vi "Calc sensitivity.vi"(7 "dB Reference":dbl=84.0, 9 "Frequency list Adjusted":T1(array[cluster])=[{"frequency [Hz]"=200.0, "amplitude [V]"=0.5}, {"frequency [Hz]"=224.0, "amplitude [V]"=0.5}, {"frequency [Hz]"=250.0, "amplitude [V]"=0.5}, {"frequency [Hz]"=280.0, "amplitude [V]"=0.5}, {"frequency [Hz]"=315.0, "amplitude [V]"=0.5}, {"frequency [Hz]"=355.0, "amplitude [V]"=0.5}, {"frequency [Hz]"=400.0, "amplitude [V]"=0.5}, {"frequency [Hz]"=450.0, "amplitude [V]"=0.5}, {"frequency [Hz]"=500.0, "amplitude [V]"=0.5}, {"frequency [Hz]"=560.0, "amplitude [V]"=0.5}, {"frequency [Hz]"=630.0, "amplitude [V]"=0.5}, {"frequency [Hz]"=710.0, "amplitude [V]"=0.5}, {"frequency [Hz]"=800.0, "amplitude [V]"=0.5}, {"frequency [Hz]"=900.0, "amplitude [V]"=0.5}, {"frequency [Hz]"=1000.0, "amplitude [V]"=0.5}, {"frequency [Hz]"=1120.0, "amplitude [V]"=0.5}, {"frequency [Hz]"=1250.0, "amplitude [V]"=0.5}, {"frequency [Hz]"=1400.0, "amplitude [V]"=0.5}, {"frequency [Hz]"=1600.0, "amplitude [V]"=0.5}, {"frequency [Hz]"=1800.0, "amplitude [V]"=0.5}, {"frequency [Hz]"=2000.0, "amplitude [V]"=0.5}, {"frequency [Hz]"=2240.0, "amplitude [V]"=0.5}, {"frequency [Hz]"=2500.0, "amplitude [V]"=0.5}, {"frequency [Hz]"=2800.0, "amplitude [V]"=0.5}, {"frequency [Hz]"=3150.0, "amplitude [V]"=0.5}, {"frequency [Hz]"=3550.0, "amplitude [V]"=0.5}, {"frequency [Hz]"=4000.0, "amplitude [V]"=0.5}, {"frequency [Hz]"=4500.0, "amplitude [V]"=0.5}, {"frequency [Hz]"=5000.0, "amplitude [V]"=0.5}, {"frequency [Hz]"=5600.0, "amplitude [V]"=0.5}, {"frequency [Hz]"=6300.0, "amplitude [V]"=0.5}, {"frequency [Hz]"=7100.0, "amplitude [V]"=0.5}, {"frequency [Hz]"=8000.0, "amplitude [V]"=0.5}] {"amplitude [V]" format="%.6f"; "frequency [Hz]" format="%.2f"}, 10 "Frequency [Hz]":dbl, 11 "Fundamental Response":T2(graph) caption="Fundamental-Response") -> (1 "Sensitivity_Pointer":i32, 2 "Sensitivity Frequency (Hz)":dbl, 3 "Sensitivity (mV/Pa)":dbl)   [LabVIEW 2018]
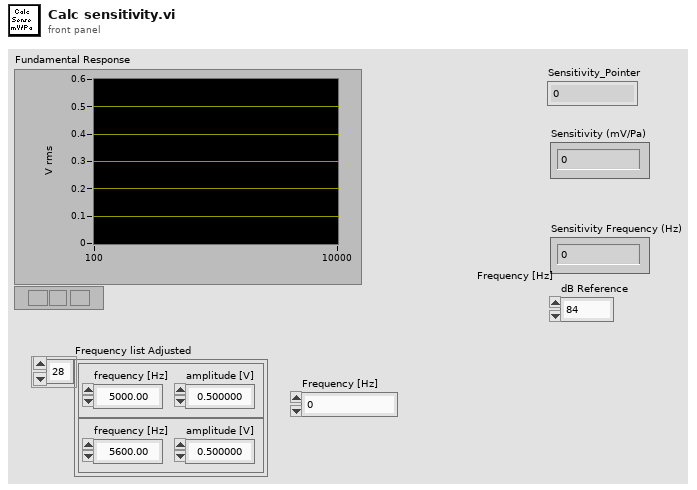
[diagram p1: front panel]
types:
  T1 = cluster{"frequency [Hz]":dbl, "amplitude [V]":dbl}[]
  T2 = cluster{"frequency [Hz]":dbl[], "amplitude":dbl[]}
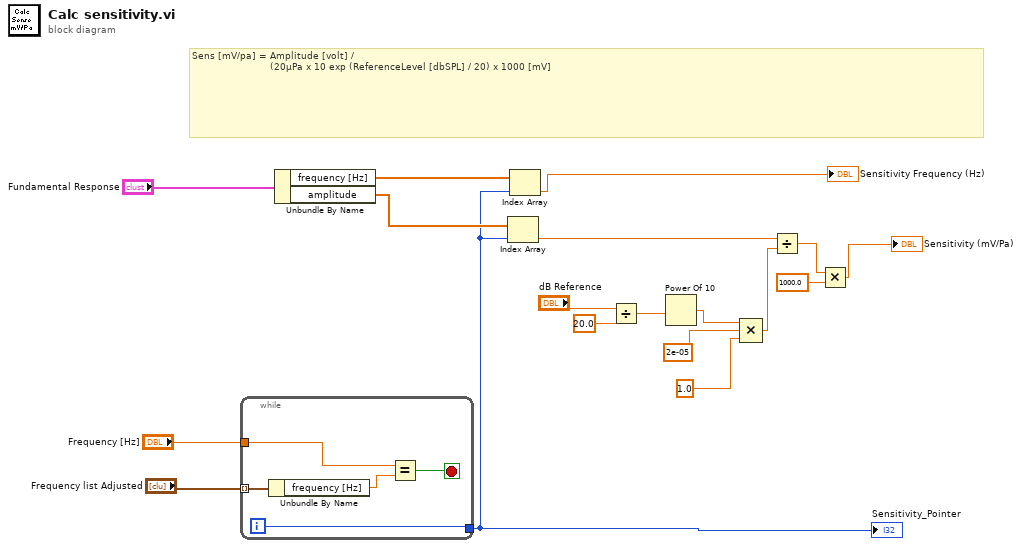
[diagram p0: block diagram]
diagram:
  # "Sens [mV/pa] = Amplitude [volt] / \n                          (20µPa x 10 exp (ReferenceLevel [dbSPL] / 20) x 1000 [mV]"
  n1 = while {
    tunnel: "Frequency list Adjusted" -> [w23] mode=indexing
    tunnel: "Frequency [Hz]" -> [w22]
    tunnel: [w19] -> w8
    i -> [w19]
    stop <- w20 stop-if-true
    n2 = Unbundle By Name(w23) -> ("frequency [Hz]"=w21:dbl)
    n3 = Equal?(x=w22, y=w21) -> (x = y?=w20:bool)
  }
  "Sensitivity_Pointer" <- w8
  n4 = Unbundle By Name("Fundamental Response") -> ("frequency [Hz]"=w7:dbl[], "amplitude"=w15:dbl[])
  n5 = Index Array(array=w15, index=w8) -> (element=w14:dbl)
  n6 = Index Array(array=w7, index=w8) -> (element=→"Sensitivity Frequency (Hz)":dbl)
  n7 = Divide(x="dB Reference", y=20.0) -> (x/y=w13:dbl)
  n8 = Power Of 10(x=w13) -> (10^x=w10:dbl)
  n9 = Compound Arithmetic op=MULTIPLY(w10, 2e-05 ("y"), 1.0 ("y")) -> (w17:dbl)
  n10 = Divide(x=w14, y=w17) -> (x/y=w3:dbl)
  n11 = Multiply(x=w3, y=1000.0) -> (x*y=→"Sensitivity (mV/Pa)":dbl)
